vi "DrawGShape.vi"(2 "name":string, 3 "contents":string) -> (0 "remaining":string, 1 "Object out":refnum<vi>)   [LabVIEW 2010]
uses:
  <vilib>/picture/3D Picture Control/NI_3D Picture Control.lvlib
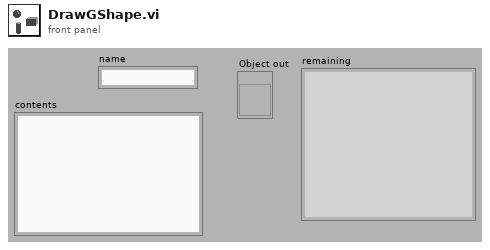
[diagram p1: front panel]
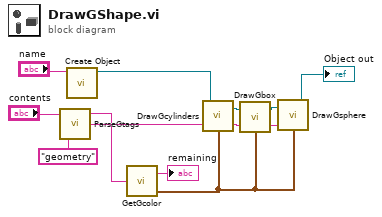
[diagram p0: block diagram]
diagram:
  n1 = call "ParseGtags.vi"("tag"="geometry", "urdf in"="contents") -> ("contents"=w5:string, "urdf out"=w3:string)  [unwired: 2 out]
  n2 = call <vilib>:"Create Object.vi"("Name"="name") -> ("Scene:New Object"=w9:refnum<vi>)  [unwired: 9 in, 1 out]
  n3 = call "GetGcolor.vi"("sdf in"=w3) -> ("color"=w1:cluster{dbl, dbl, dbl, dbl}, "sdf out"=→"remaining":string)
  n4 = call "DrawGcylinders.vi"("Object in"=w9, "Color"=w1, "contents"=w5) -> ("Object out"=w7:refnum<vi>, "remaining"=w6:string)
  n5 = call "DrawGbox.vi"("Object in"=w7, "Color"=w1, "contents"=w6) -> ("Object out"=w10:refnum<vi>, "remaining"=w11:string)
  n6 = call "DrawGsphere.vi"("Object in"=w10, "contents"=w11, "Color"=w1) -> ("Object out"=→"Object out":refnum<vi>)  [unwired: 1 out]
